vi "Motor drive globals.vi"() -> ()   [LabVIEW 2009]
panel:
  out "Piston displacement":ext format="%.2f"
  out "current motor velocity (rps)":dbl format="%.2f"
  out "Active string":string
  out "Initialize":bool
  out "Run state":bool
  out "Read string":string
  in  "Write string":string
  out "Mode":string
  in  "tic count":u32
  in  "reset":ext format="%.6f"
  out "current actual displacement rate":ext format="%.2f"
  out "internal force gauge (v)":ext format="%.6f"
  out "current selected displacement rate":string
  # "value for constant load"
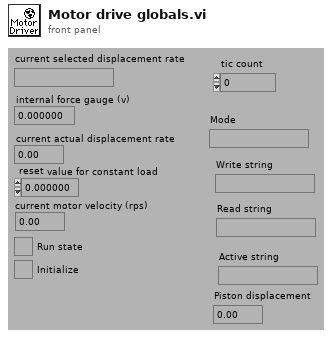
[diagram p1: front panel]
diagram:
